vi "GalvosClose.vi"(8 "error in (no error)":errorcluster, 11 "Microscope in":refnum<class "Microscope.lvclass">) -> (0 "error out":errorcluster, 3 "Microscope out":refnum<class "Microscope.lvclass">)   [LabVIEW 2012, in "Microscope.lvclass"]
uses:
  classes/Microscope.lvclass
  classes/Microscope.lvclass/Microscope.ctl
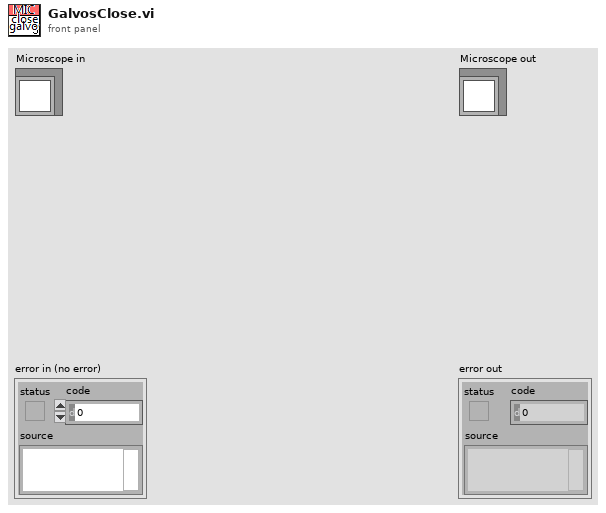
[diagram p1: front panel]
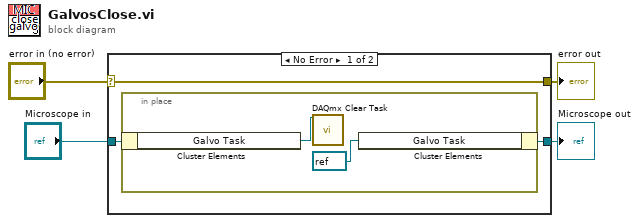
[diagram p0: block diagram]
diagram:
  n1 = case shown="No Error" "error in (no error)" {
    selector: "error in (no error)" -> [w7 w11]
    tunnel: [w7 w11] -> w3
    tunnel: [w5 w10] -> w1
    tunnel: "Microscope in" -> [w6 w10]
    frame No Error {
      n2 = in-place {
        n3 = in-place-cluster #1(w6) -> ("Galvo Task"=w8:refnum<k21>)
        n4 = call <vilib>:"DAQmx Clear Task.vi"("task in"=w8) -> ()  [unwired: 14 in, 1 out]
        n5 = in-place-cluster #1("Galvo Task"=refnum<k21> refnum ("Hardware Settings.Galvo Task")) -> (w5:refnum<class "Microscope.lvclass">)
      }
    }
    frame Error {
    }
  }
  "error out" <- w3
  "Microscope out" <- w1
